vi "is abstract node.vi"(8 "error in":errorcluster, 11 "TBM Configuration Node in":refnum<class "TBM Configuration Node.lvclass">) -> (0 "error out":errorcluster, 2 "abstract":bool, 3 "TBM Configuration Node out":refnum<class "TBM Configuration Node.lvclass">)   [LabVIEW 2013, in "PL Framework Configuration Tool.lvlib" / "TBM Configuration Node.lvclass"]
doc: "Indicates if a node is abstract. This is used for categorization during loading."
uses:
  TBM Configuration Node.lvclass
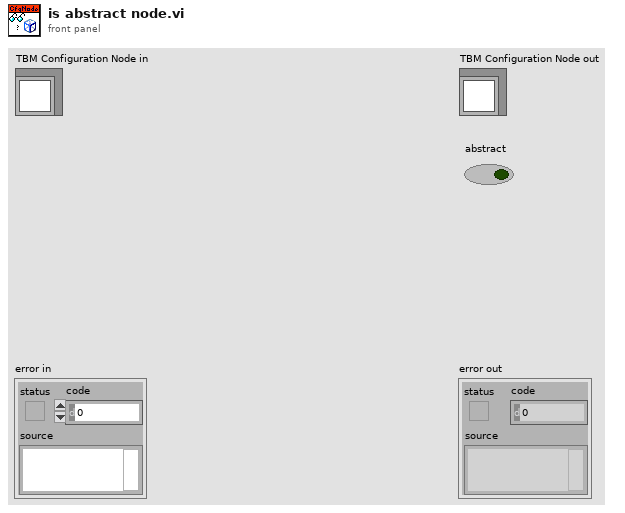
[diagram p1: front panel]
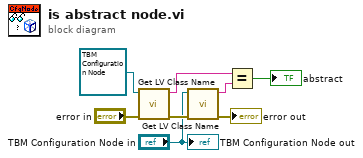
[diagram p0: block diagram]
diagram:
  n1 = call <vilib>:"Get LV Class Name.vi"("error in (no error)"="error in", "object"=refnum<class "TBM Configuration Node.lvclass"> refnum ("PL Framework Configuration Tool.lvlib:TBM Configuration Node")) -> ("error out"=w5:errorcluster, "class name"=w3:string)  [unwired: 8 in]
  n2 = call <vilib>:"Get LV Class Name.vi"("error in (no error)"=w5, "object"="TBM Configuration Node in") -> ("error out"=→"error out":errorcluster, "class name"=w2:string)  [unwired: 8 in]
  n3 = Equal?(x=w3, y=w2) -> (x = y?=→"abstract":bool)
  "TBM Configuration Node out" <- "TBM Configuration Node in"
